vi "CreateTracker.vi"(1 "height":u32, 2 "width":u32) -> (0 "return type":u64)   [LabVIEW 2011]
uses:
  cudatrack-debug.dll
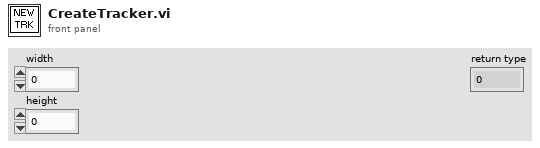
[diagram p1: front panel]
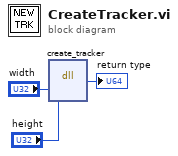
[diagram p0: block diagram]
diagram:
  n1 = dll-call lib="D:/jcnossen1/cudaqi-tracker/cudatrack/cudatrack-debug.dll" fn="create_tracker"("width"="width", "height"="height") -> ("return type"=→"return type":u64)  [unwired: 5 in, 2 out]
